vi "sv_Get IMD Frequencies (Multitone).vi"(7 "harmonic frequencies [Hz]":dbl[](array[numeric]), 9 "maximum order":u8=3, 10 "frequency range [Hz]":cluster{"start":dbl, "stop":dbl}={"start"=20.0, "stop"=20000.0}, 11 "reference tones":T1(array[cluster])) -> (3 "intermodulation frequencies":dbl[](array[numeric]))   [LabVIEW 2017, in "SoundVib_Distortion.lvlib"]
uses:
  <vilib>/addons/Sound and Vibration/svt_Distortion/SoundVib_Distortion.lvlib
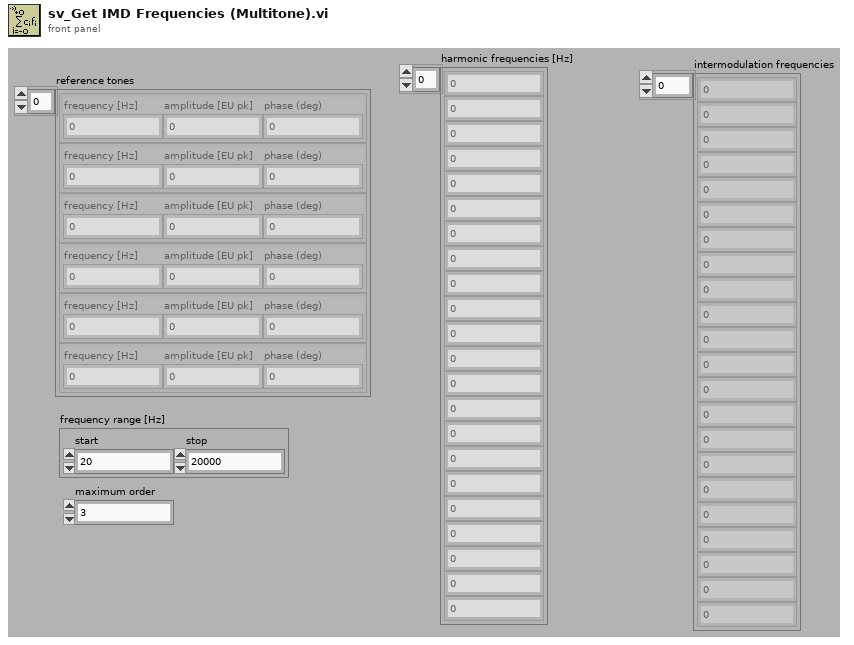
[diagram p1: front panel]
types:
  T1 = cluster{"frequency [Hz]":dbl, "amplitude [EU pk]":dbl, "phase (deg)":dbl}[]
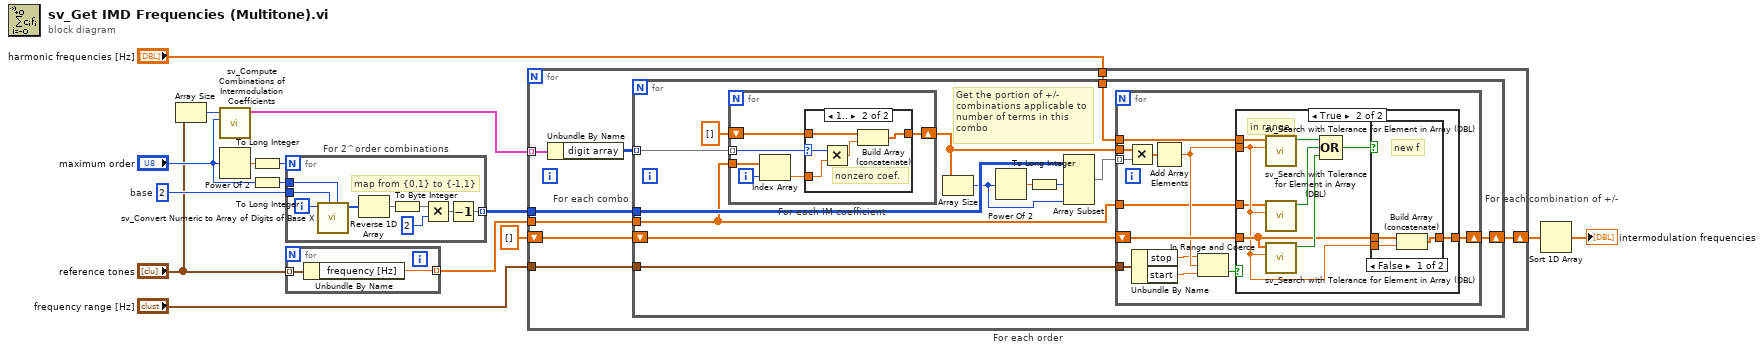
[diagram p0: block diagram]
diagram:
  w11 = u8 2  # base
  n1 = Array Size(array="reference tones") -> (size(s)=w4:i32)
  n2 = call <vilib>:"sv_Compute Combinations of Intermodulation Coefficients.vi"("maximum order"="maximum order", "number of tones"=w4) -> ("intermodulation coefficients"=w9:cluster{"order":i32, "digit array":u8[][]}[])  [unwired: 9 in]
  n3 = Power Of 2(x="maximum order") -> (2^x=w5:dbl)
  n4 = To Long Integer(number=w5) -> (32bit integer=w6:i32)
  n5 = To Long Integer(number="maximum order") -> (32bit integer=w8:i32)
  n6 = for "For 2^order combinations" {
    N: w6 -> [_]
    tunnel: w8 -> [w24]
    tunnel: [w17] -> w10 mode=indexing
    tunnel: w11 -> [w16]
    i -> [w23]
    # "map from {0,1} to {-1,1}"
    n7 = call <vilib>:"sv_Convert Numeric to Array of Digits of Base X.vi"("fixed width"=w24, "base"=w16, "numeric"=w23) -> ("byte array"=w22:u8[])  [unwired: 8 in]
    n8 = Reverse 1D Array(array=w22) -> (reversed array=w21:u8[])
    n9 = To Byte Integer(number=w21) -> (8bit integer=w20:i8[])
    n10 = Multiply(x=w20, y=i8 2 ("base")) -> (x*y=w19:i8[])
    n11 = Decrement(x=w19) -> (x-1=w17:i8[])
  }
  n12 = for {
    tunnel: "reference tones" -> [w26] mode=indexing
    tunnel: [w25] -> w2 mode=indexing
    n13 = Unbundle By Name(w26) -> ("frequency [Hz]"=w25:dbl)
  }
  n14 = for "For each order" {
    tunnel: w9 -> [w34] mode=indexing
    tunnel: w10 -> [w32]
    tunnel: w2 -> [w31]
    shift-right: [w28] -> w15
    shift-left: dbl[] [] -> [w29]
    tunnel: "harmonic frequencies [Hz]" -> [w30]
    tunnel: "frequency range [Hz]" -> [w27]
    n15 = Unbundle By Name(w34) -> ("digit array"=w33:u8[][])
    n16 = for "For each combo" {
      tunnel: w33 -> [w44] mode=indexing
      tunnel: w32 -> [w47]
      tunnel: w31 -> [w37]
      tunnel: w30 -> [w41]
      shift-right: [w39] -> w28
      shift-left: w29 -> [w40]
      tunnel: w27 -> [w38]
      # "Get the portion of +/- combinations applicable to number of terms in this combo"
      n17 = for "For each IM coefficient" {
        tunnel: w44 -> [w52] mode=indexing
        shift-right: [w53] -> w42
        shift-left: dbl[] [] -> [w51]
        tunnel: w37 -> [w50]
        i -> [w49]
        n18 = Index Array(array=w50, index=w49) -> (element=w48:dbl)
        n19 = case shown="1.." w52 {
          selector: w52 -> [_ w57]
          tunnel: [w54 w59] -> w53
          tunnel: w51 -> [w54 w58]
          tunnel: w48 -> [_ w55]
          frame 0, Default {
          }
          frame 1.. {
            # "nonzero coef."
            n20 = Multiply(x=w57, y=w55) -> (x*y=w56:dbl)
            n21 = Build Array (concatenate)(w58, w56) -> (w59:dbl[])
          }
        }
      }
      n22 = Array Size(array=w42) -> (size(s)=w35:i32)
      n23 = Power Of 2(x=w35) -> (2^x=w46:dbl)
      n24 = To Long Integer(number=w46) -> (32bit integer=w36:i32)
      n25 = Array Subset(array=w47, length (row)=w36, length (col)=w35) -> (w45:i8[][])  [unwired: 2 in]
      n26 = for "For each combination of +/-" {
        tunnel: w45 -> [w70] mode=indexing
        tunnel: w42 -> [w71]
        tunnel: w41 -> [w68]
        shift-right: [w64] -> w39
        shift-left: w40 -> [w67]
        tunnel: w38 -> [w63]
        tunnel: w37 -> [w60]
        n27 = Multiply(x=w71, y=w70) -> (x*y=w69:dbl[])
        n28 = Unbundle By Name(w63) -> ("stop"=w62:dbl, "start"=w61:dbl)
        n29 = Add Array Elements(numeric array=w69) -> (sum=w66:dbl)
        n30 = In Range and Coerce(upper limit=w62, x=w66, lower limit=w61) -> (In Range?=w65:bool)  [unwired: 1 out]
        n31 = case shown="True" w65 {
          tunnel: w68 -> [_ w81]
          tunnel: w67 -> [w72 w77]
          tunnel: w66 -> [_ w75]
          tunnel: [w72 w76] -> w64
          tunnel: w60 -> [_ w73]
          frame False {
            # "not in range"
          }
          frame True {
            # "in range"
            n32 = call <vilib>:"sv_Search with Tolerance for Element in Array (DBL).vi"("element"=w75, "1D array"=w81) -> ("found?"=w80:bool)  [unwired: 7 in, 2 out]
            n33 = call <vilib>:"sv_Search with Tolerance for Element in Array (DBL).vi"("element"=w75, "1D array"=w73) -> ("found?"=w74:bool)  [unwired: 7 in, 2 out]
            n34 = call <vilib>:"sv_Search with Tolerance for Element in Array (DBL).vi"("element"=w75, "1D array"=w77) -> ("found?"=w79:bool)  [unwired: 7 in, 2 out]
            n35 = Compound Arithmetic op=OR(w80, w74, w79) -> (w78:bool)
            n36 = case shown="False" w78 {
              tunnel: w77 -> [w84 w85]
              tunnel: [w83 w85] -> w76
              tunnel: w75 -> [w82 _]
              frame False {
                # "new f"
                n37 = Build Array (concatenate)(w84, w82) -> (w83:dbl[])
              }
              frame True {
                # "duplicate"
              }
            }
          }
        }
      }
    }
  }
  n38 = Sort 1D Array(array=w15) -> (sorted array=→"intermodulation frequencies":dbl[])
